vi "Joystick-avg.vi"(8 "Joystic right axis in":dbl format="%#_13g", 11 "Joystic left axis in":dbl format="%#_13g") -> (0 "Right out":dbl, 3 "Left out":dbl)   [LabVIEW 2015]
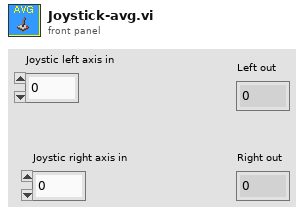
[diagram p1: front panel]
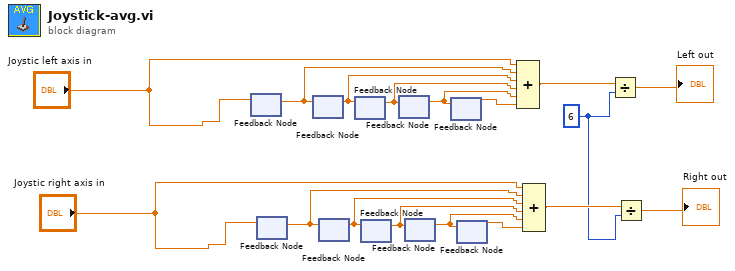
[diagram p0: block diagram]
diagram:
  w1 = 6
  n1 = feedback #1() -> (w16:dbl)  [unwired: 1 in]
  n2 = feedback-in #1("Joystic left axis in") -> ()
  n3 = feedback #2() -> (w8:dbl)  [unwired: 1 in]
  n4 = feedback-in #2("Joystic right axis in") -> ()
  n5 = feedback #3() -> (w15:dbl)  [unwired: 1 in]
  n6 = feedback-in #3(w16) -> ()
  n7 = feedback #4() -> (w7:dbl)  [unwired: 1 in]
  n8 = feedback-in #4(w8) -> ()
  n9 = feedback #5() -> (w14:dbl)  [unwired: 1 in]
  n10 = feedback-in #5(w15) -> ()
  n11 = feedback #6() -> (w6:dbl)  [unwired: 1 in]
  n12 = feedback-in #6(w7) -> ()
  n13 = feedback #7() -> (w13:dbl)  [unwired: 1 in]
  n14 = feedback-in #7(w14) -> ()
  n15 = feedback #8() -> (w5:dbl)  [unwired: 1 in]
  n16 = feedback-in #8(w6) -> ()
  n17 = feedback #9() -> (w12:dbl)  [unwired: 1 in]
  n18 = feedback-in #9(w13) -> ()
  n19 = feedback #10() -> (w4:dbl)  [unwired: 1 in]
  n20 = feedback-in #10(w5) -> ()
  n21 = Compound Arithmetic op=ADD("Joystic left axis in", w16, w15, w14, w13, w12) -> (w11:dbl)
  n22 = Compound Arithmetic op=ADD("Joystic right axis in", w8, w7, w6, w5, w4) -> (w3:dbl)
  n23 = Divide(x=w11, y=w1) -> (x/y=→"Left out":dbl)
  n24 = Divide(x=w3, y=w1) -> (x/y=→"Right out":dbl)
